vi "Add Required Status Channels.vi"(8 "error in":errorcluster, 11 "custom device ref":T1 format="%.0x") -> (0 "error out":errorcluster, 2 "status section ref":T1 format="%.0x", 3 "custom device ref out":T1 format="%.0x")   [LabVIEW 2020, in "Ballard ARINC 429 Scripting.lvlib"]
doc: "Adds 'Status' section and required channels including error status channels and asynchronous loop time."
uses:
  Ballard ARINC 429 Scripting.lvlib
  <vilib>/NI VeriStand/Custom Device API/Custom Device Item Ref.ctl
  <vilib>/NI VeriStand/Custom Device API/Custom Device API.lvlib
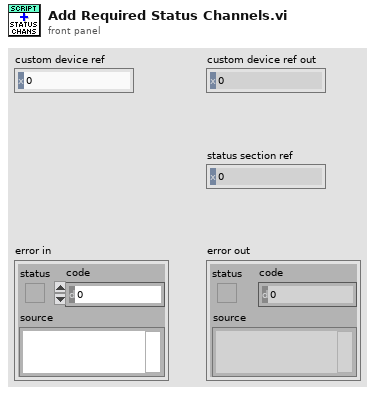
[diagram p1: front panel]
types:
  T1 = typedef "Custom Device API.lvlib/Custom Device Item Ref.ctl" = u64
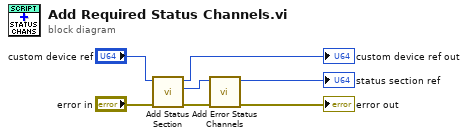
[diagram p0: block diagram]
diagram:
  n1 = call "Add Status Section.vi"("error in"="error in", "custom device ref"="custom device ref") -> ("error out"=w4:errorcluster, "status ref"=w7:T1, "custom device ref out"=→"custom device ref out":T1)  [unwired: 7 in]
  n2 = call "Add Error Status Channels.vi"("error in"=w4, "status section ref"=w7) -> ("error out"=→"error out":errorcluster, "status section ref out"=→"status section ref":T1)  [unwired: 8 in]
